vi "Panel Output Voltage Test.vi"(7 "Socket Index":i32, 11 "DMM In":string) -> (0 "error out":errorcluster, 3 "Voltage":dbl)   [LabVIEW 2013]
doc: "Measure the voltage produced by the solar panel after setting the ambient lighting and temperature conditions."
uses:
  Exercises/Driver Simulation API/Support/DMM/Signal Types.ctl
  Exercises/Driver Simulation API/Support/DMM.lvlib
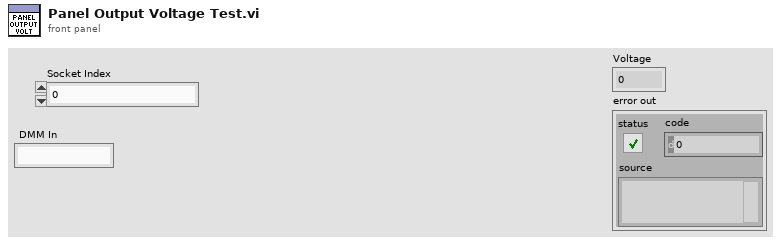
[diagram p1: front panel]
types:
  T1 = typedef "Driver Simulation.lvlib/DMM.lvlib/Signal Types.ctl" = enum16{"DC", "AC"}
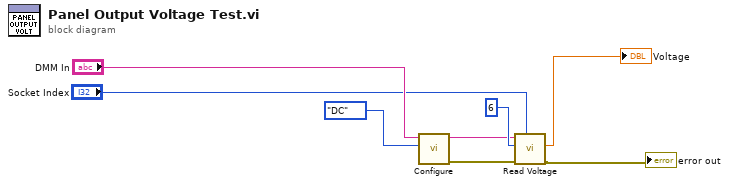
[diagram p0: block diagram]
diagram:
  n1 = call "Configure.vi"("signalType"=Signal_Types."DC", "DMM in"="DMM In") -> ("error out"=w3:errorcluster, "DMM out"=w5:string)  [unwired: 8 in]
  n2 = call "Read Voltage.vi"("Test Socket (0)"="Socket Index", "error in (no error)"=w3, "Channel"=6, "DMM in"=w5) -> ("error out"=→"error out":errorcluster, "Voltage"=→"Voltage":dbl)  [unwired: 5 in, 1 out]
